vi "Get List of Properties by level.vi"(7 "UserName":string="jimbo", 8 "error in (no error)":errorcluster, 11 "eSearch Types":T1=enum."eSearchChannelGroup") -> (0 "error out":errorcluster, 1 "Number Found":i32, 2 "Data Returned?":bool, 3 "Unique Name List":string[](array[string]))   [LabVIEW 2011]
uses:
  eSearch Types.ctl
  DataFinder Comparisons.ctl
  Datafinder Query.ctl
  DD/lib/Query Queue.ctl
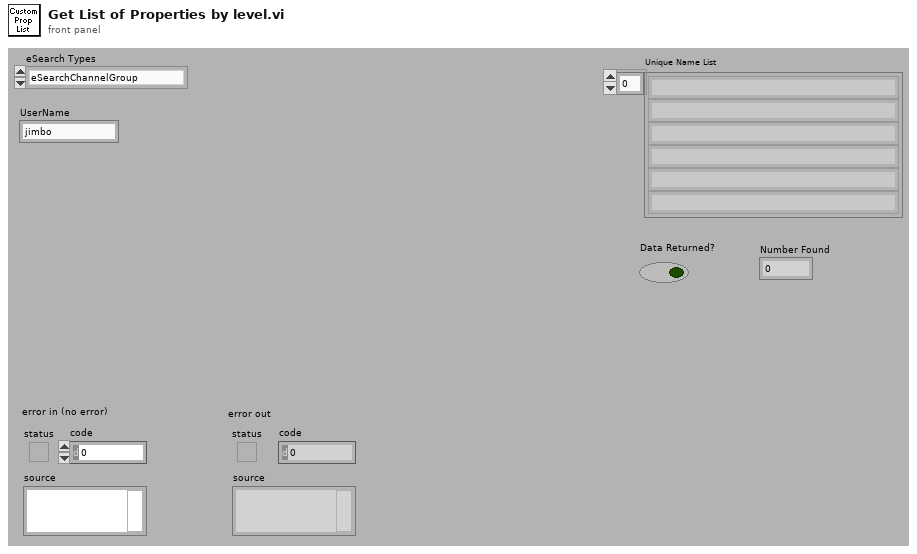
[diagram p1: front panel]
types:
  T1 = typedef "eSearch Types.ctl" = enum16{"eSearchFile", "eSearchChannelGroup", "eSearchChannel"}
  T2 = typedef "Query Queue.ctl" = cluster{"UserName":string, "Search Parameters":T3[], "eSearch Type":T1, "Query Name (vbs)":string, "Response queue name":string, "Logic String":string}
  T3 = typedef "Datafinder Query.ctl" = cluster{"eSearch Types":T1, "Property Name":string, "DataFinder Comparisons":T4, "Property Value":string}
  T4 = typedef "DataFinder Comparisons.ctl" = enum16{"=", "<>", "<", "<=", ">", ">="}
  T5 = typedef "DIAdem Query Result.ctl" = cluster{"Results":string[][], "# of Items":i32, "Data Returned?":bool, "Result TDM":path, "Timed Out?":bool}
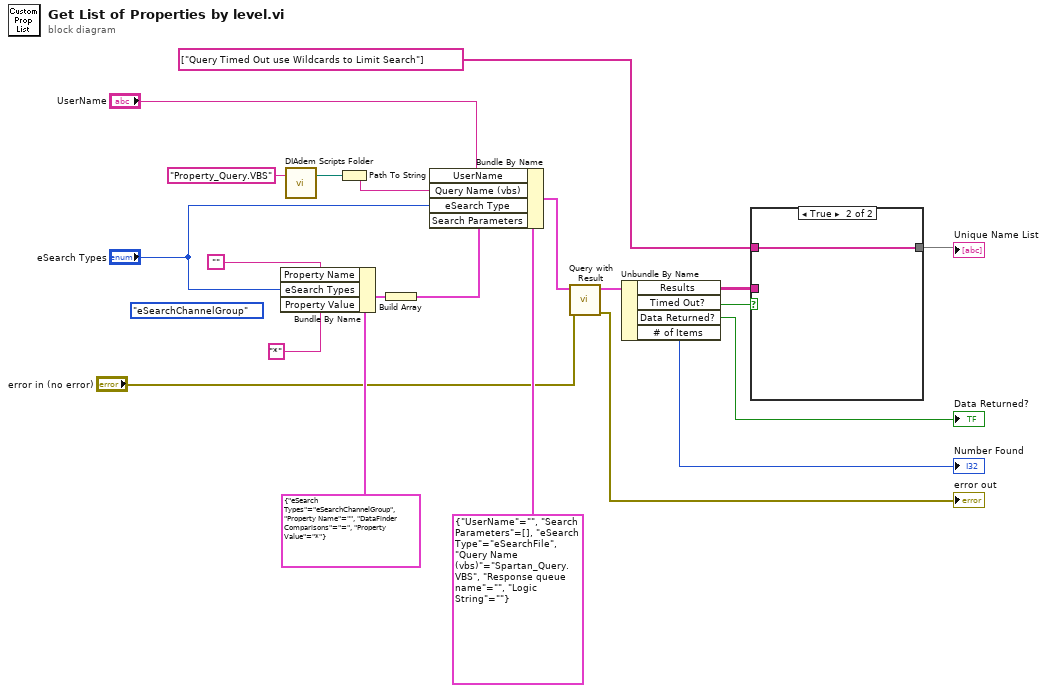
[diagram p0: block diagram]
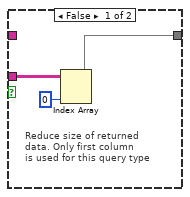
[diagram p2: hidden frame]
diagram:
  (unwired) eSearch_Types."eSearchChannelGroup" ("eSearch Types")
  n1 = Bundle By Name(cluster=T3 {"eSearch Types"=enum."eSearchChannelGroup", "Property Name"="", "DataFinder Comparisons"=enum."=", "Property Value"="*"} ("Data Finder Parameters"), "Property Name"="", "eSearch Types"="eSearch Types", "Property Value"="*") -> (w19:T3)
  n2 = call "DIAdem Scripts Folder.vi"("Relative Path (\"\" - Folder)"="Property_Query.VBS" ("Query Name.vbs")) -> ("Scripts Folder"=w16:path)  [unwired: 2 out]
  n3 = Path To String(path=w16) -> (string=w1:string)
  n4 = Build Array(w19) -> (w4:T3[])
  n5 = Bundle By Name(cluster=T2 {"UserName"="", "Search Parameters"=[], "eSearch Type"=enum."eSearchFile", "Query Name (vbs)"="Spartan_Query.VBS", "Response queue name"="", "Logic String"=""} ("Query Parameter Data"), "UserName"="UserName", "Query Name (vbs)"=w1, "eSearch Type"="eSearch Types", "Search Parameters"=w4) -> (w5:T2)
  n6 = call "Query with Result.vi"("error in (no error)"="error in (no error)", "Query Parameter Data"=w5) -> ("error out"=→"error out":errorcluster, "Query Return Data"=w18:T5)  [unwired: 3 in, 5 out]
  n7 = Unbundle By Name(w18) -> ("Results"=w11:string[][], "Timed Out?"=w10:bool, "Data Returned?"=→"Data Returned?":bool, "# of Items"=→"Number Found":i32)
  n8 = case shown="True" w10 {
    tunnel: w11 -> [w24 _]
    tunnel: [w22 w25] -> w20
    tunnel: string[] ["Query Timed Out use Wildcards to Limit Search"] ("Results") -> [_ w25]
    frame False {
      # "Reduce size of returned data. Only first column\nis used for this query type"
      n9 = Index Array(array=w24, index (col)=0 ("disabled index (col)")) -> (element=w22:string[])  [unwired: 1 in]
    }
    frame True {
    }
  }
  "Unique Name List" <- w20
